vi "Wave1D_Cal AU.vi"(10 "A":T2, 11 "U":dbl[](array[numeric])) -> (0 "error":i32, 3 "AU":dbl[](array[numeric]))   [LabVIEW 2017, in "NI_PDE.lvlib"]
uses:
  <vilib>/gmath/NI_PDE.lvlib
  <vilib>/Analysis/Matrix/Datatypes/RealMatrix.ctl
  <vilib>/Analysis/baseanly.llb/A x Vector.vi
  <vilib>/Analysis/NI_AALBase.lvlib
  <vilib>/Analysis/Matrix/NI_Matrix.lvlib
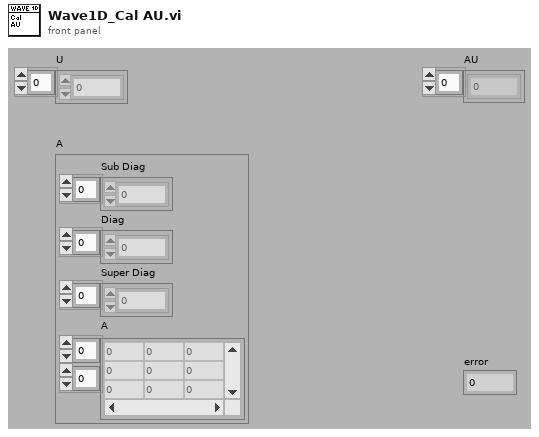
[diagram p1: front panel]
types:
  T1 = typedef "NI_Matrix.lvlib/RealMatrix.ctl" = dbl[][]
  T2 = cluster{"Sub Diag":dbl[], "Diag":dbl[], "Super Diag":dbl[], "A":T1}
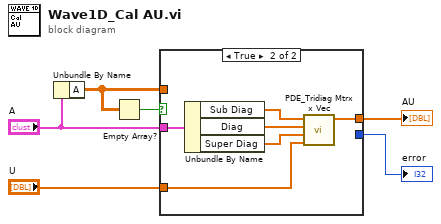
[diagram p0: block diagram]
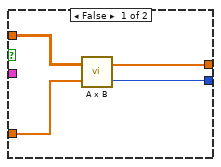
[diagram p2: hidden frame]
diagram:
  n1 = Unbundle By Name("A") -> ("A"=w4:T1)
  n2 = Empty Array?(array=w4) -> (empty?=w6:bool)
  n3 = case shown="True" w6 {
    tunnel: "U" -> [w9 w12]
    tunnel: w4 -> [w10 _]
    tunnel: [w8 w11] -> w3
    tunnel: [w7 _] -> w1
    tunnel: "A" -> [_ w16]
    frame False {
      n4 = call-poly <vilib>:"A x B.vi"("Vector"=w9, "A"=w10) -> ("error"=w7:i32, "A x Vector"=w8:dbl[])
    }
    frame True {
      n5 = Unbundle By Name(w16) -> ("Sub Diag"=w15:dbl[], "Diag"=w14:dbl[], "Super Diag"=w13:dbl[])
      n6 = call <vilib>:"PDE_Tridiag Mtrx x Vec.vi"("X"=w12, "Super Diag"=w13, "Diag"=w14, "Sub Diag"=w15) -> ("Mtrx x X"=w11:dbl[])  [unwired: 7 out]
    }
  }
  "AU" <- w3
  "error" <- w1
